vi "Panel Resized.vi"(6 "Sizing Refnums":T2, 8 "error in (no error)":errorcluster, 9 "Origin":cluster{"H":i16, "V":i16}, 10 "NewBnds":T1, 11 "Size Constraints":cluster{"min tab width":i32, "w/h":dbl}) -> (0 "error out":errorcluster)   [LabVIEW 2016]
uses:
  <vilib>/Utility/miscctls.llb/LVRectTypeDef.ctl
  <vilib>/Utility/miscctls.llb/LVRowAndColumnTypeDef.ctl
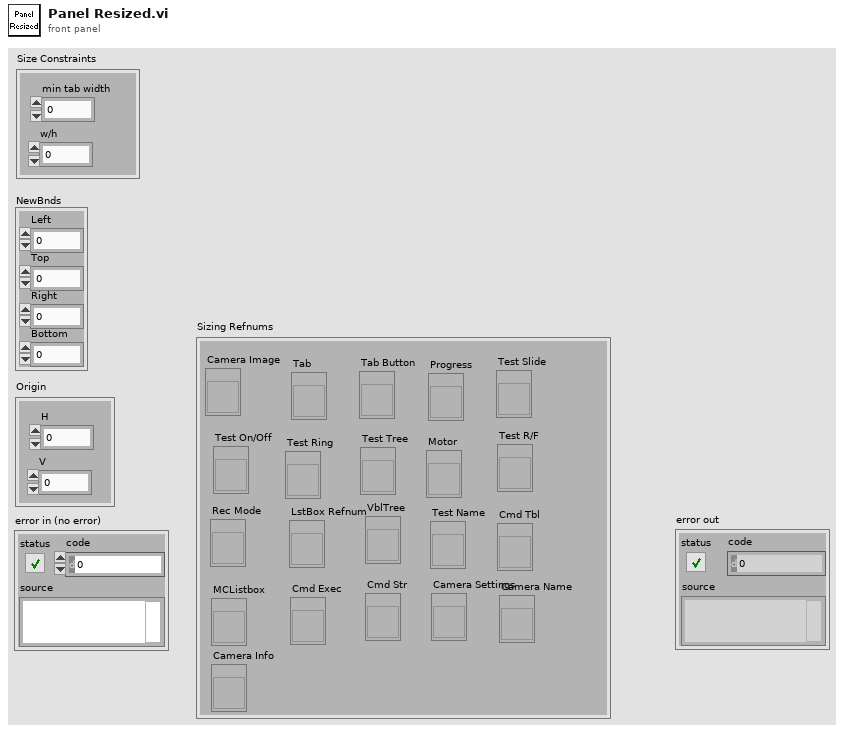
[diagram p1: front panel]
types:
  T1 = typedef "LVRectTypeDef.ctl" = cluster{"Left":i16, "Top":i16, "Right":i16, "Bottom":i16}
  T2 = cluster{"Camera Image":refnum<vi>, "Tab":refnum<vi>, "Tab Button":refnum<vi>, "Rec Mode":refnum<vi>, "Test Slide":refnum<vi>, "Test On/Off":refnum<vi>, "Test Ring":refnum<vi>, "Test R/F":refnum<vi>, "Test Name":refnum<vi>, "Motor":refnum<vi>, "Progress":refnum<vi>, "LstBox Refnum":refnum<vi>, "Test Tree":refnum<vi>, "VblTree":refnum<vi>, "Cmd Tbl":refnum<vi>, "MCListbox":refnum<vi>, "Cmd Exec":refnum<vi>, "Cmd Str":refnum<vi>, "Camera Settings":refnum<vi>, "Camera Name":refnum<vi>, "Camera Info":refnum<vi>}
  T3 = typedef "LVRowAndColumnTypeDef.ctl" = cluster{"Row":i32, "Column":i32}
  T4 = typedef "LVPositionTypeDef.ctl" = cluster{"Left":i32, "Top":i32}
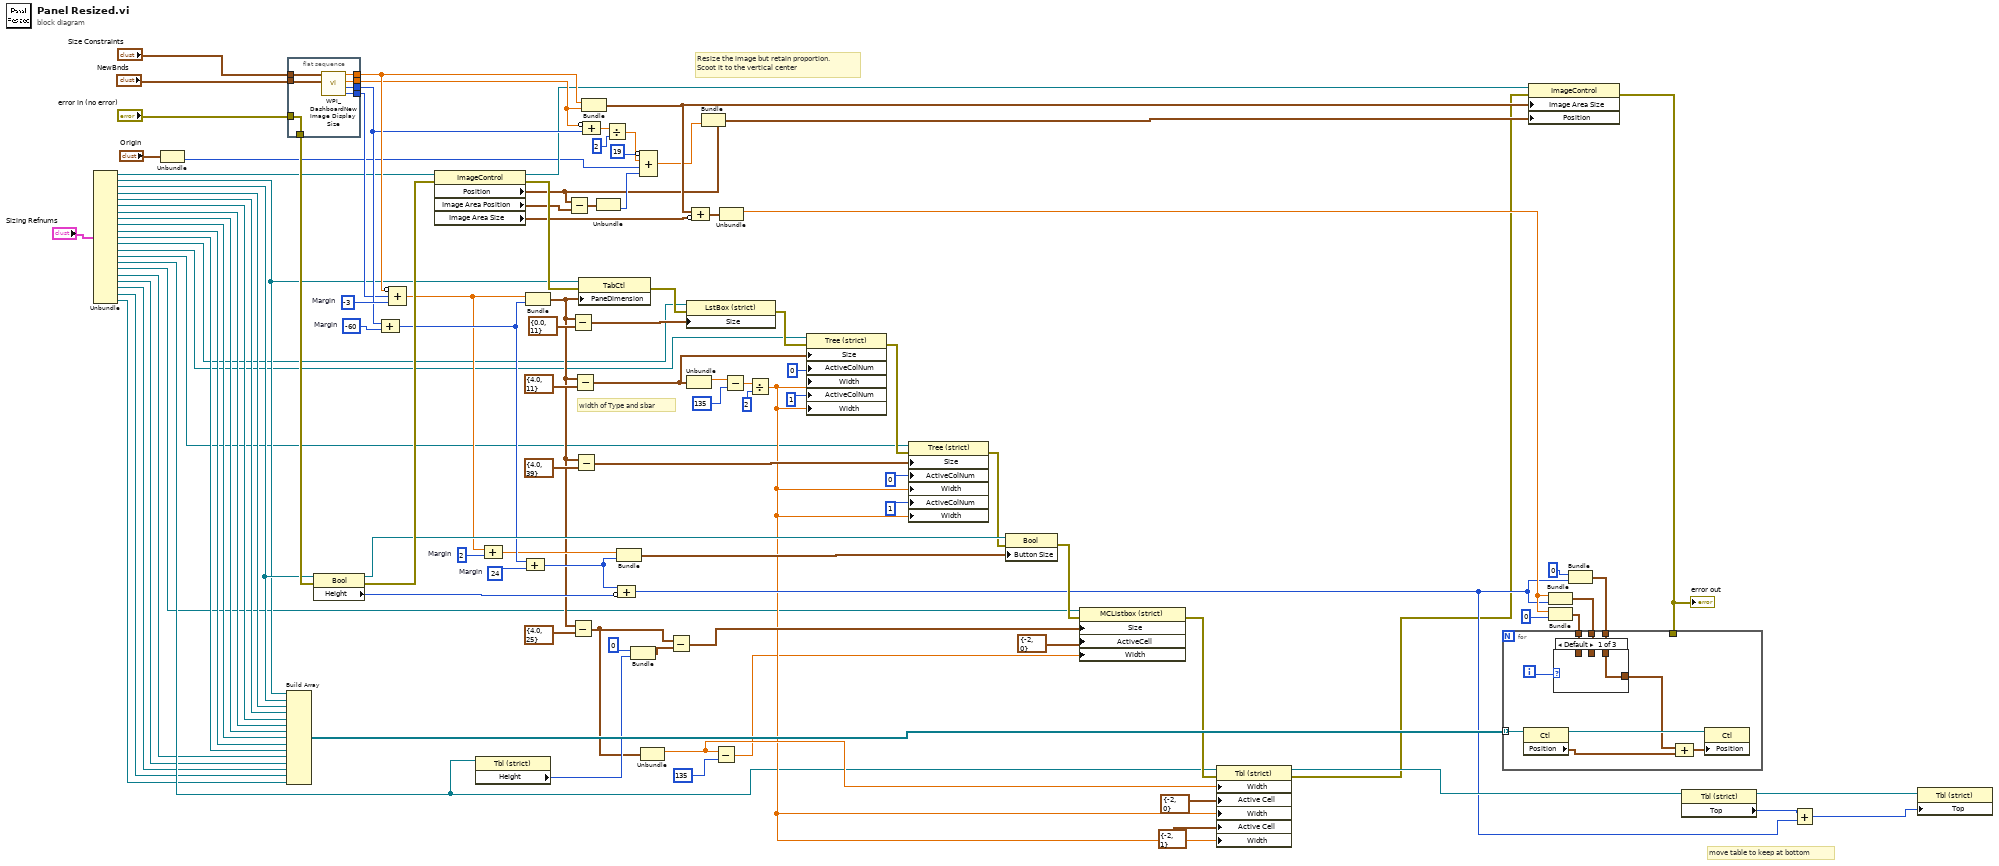
[diagram p0: block diagram]
diagram:
  w94 = 24  # Margin
  w92 = 2  # Margin
  w88 = -60  # Margin
  w98 = -3  # Margin
  # "move table to keep at bottom"
  # "width of Type and sbar"
  # "Resize the image but retain proportion.\nScoot it to the vertical center"
  n1 = Unbundle("Sizing Refnums") -> ("Camera Image"=w62:refnum<vi>, "Tab"=w63:refnum<vi>, "Tab Button"=w71:refnum<vi>, "Rec Mode"=w18:refnum<vi>, "Test Slide"=w17:refnum<vi>, "Test On/Off"=w16:refnum<vi>, "Test Ring"=w15:refnum<vi>, "Test R/F"=w14:refnum<vi>, "Test Name"=w13:refnum<vi>, "Motor"=w12:refnum<vi>, "Progress"=w11:refnum<vi>, "LstBox Refnum"=w10:refnum<vi>, "Test Tree"=w9:refnum<vi>, "VblTree"=w8:refnum<vi>, "Cmd Tbl"=w7:refnum<vi>, "MCListbox"=w6:refnum<vi>, "Cmd Exec"=w5:refnum<vi>, "Cmd Str"=w4:refnum<vi>, "Camera Settings"=w3:refnum<vi>, "Camera Name"=w2:refnum<vi>, "Camera Info"=w1:refnum<vi>)
  n2 = Unbundle("Origin") -> ("V"=w68:i16)  [unwired: 1 out]
  n3 = Build Array(w63, w71, w18, w17, w16, w15, w14, w13, w12, w11, w5, w4, w3, w2, w1) -> (w107:refnum<vi>[])
  n4 = flat-sequence {
    tunnel: "NewBnds" -> [w114]
    tunnel: "Size Constraints" -> [w113]
    tunnel: [w112] -> w87
    tunnel: [w111] -> w95
    tunnel: [w110] -> w96
    tunnel: [w109] -> w97
    tunnel: [w108] -> w106
    tunnel: "error in (no error)" -> [w108]
    frame #0 {
      n5 = call <vilib>:"WPI_DashboardNew Image Display Size.vi"("NewBnds"=w114, "Size Constraints"=w113) -> ("Window Width"=w112:i16, "Window Height"=w110:i16, "Height"=w111:dbl, "Width"=w109:dbl)  [unwired: 6 in]
    }
  }
  n6 = property class="Bool"(reference=w71, error in=w106) -> (reference out=w101:refnum<vi>, error out=w105:errorcluster, "Height"=w100:u32)
  n7 = Compound Arithmetic op=unknown(w96, w88) -> (w93:i32)
  n8 = Compound Arithmetic op=ADD(invert w97, w87, w98) -> (w91:dbl)
  n9 = property class="ImageControl"(reference=w62, error in=w105) -> (reference out=w80:refnum<vi>, error out=w104:errorcluster, "Position"=w79:T4, "Image Area Position"=w74:cluster{"Left":i32, "Top":i32}, "Image Area Size"=w85:cluster{"Width":u32, "Height":u32})
  n10 = property class="Tbl (strict)"(reference=w7) -> ("Height"=w37:u32)  [unwired: 1 in, 2 out]
  n11 = Compound Arithmetic op=ADD(w91, w92) -> (w90:dbl)
  n12 = Bundle(w91, w93) -> (w32:cluster{dbl, i32})  [unwired: 1 in]
  n13 = Compound Arithmetic op=ADD(w93, w94) -> (w99:i32)
  n14 = Subtract(x=w79, y=w74) -> (x-y=w81:T4)
  n15 = Subtract(x=w32, y=cluster{dbl, i32} {0.0, 11}) -> (x-y=w60:cluster{dbl, i32})
  n16 = Subtract(x=w32, y=cluster{dbl, i32} {4.0, 25}) -> (x-y=w34:cluster{dbl, i32})
  n17 = Subtract(x=w32, y=cluster{dbl, i32} {4.0, 11}) -> (x-y=w50:cluster{dbl, i32})
  n18 = Subtract(x=w32, y=cluster{dbl, i32} {4.0, 39}) -> (x-y=w56:cluster{dbl, i32})
  n19 = property class="TabCtl"(reference=w63, error in=w104, "PaneDimension"=w32) -> (error out=w61:errorcluster)  [unwired: 1 out]
  n20 = Bundle("Width"=w97, "Height"=w95) -> (w83:cluster{"Width":dbl, "Height":dbl})  [unwired: 1 in]
  n21 = Compound Arithmetic op=ADD(invert w95, w96) -> (w75:dbl)
  n22 = Unbundle(w81) -> ("Top"=w82:i32)  [unwired: 1 out]
  n23 = Divide(x=w75, y=2) -> (x/y=w77:dbl)
  n24 = Bundle(w90, w99) -> (w89:cluster{dbl, i32})  [unwired: 1 in]
  n25 = Compound Arithmetic op=ADD(w99, invert w100) -> (w28:u32)
  n26 = Bundle(0, "Height"=w37) -> (w35:cluster{i32, "Height":u32})  [unwired: 1 in]
  n27 = Compound Arithmetic op=ADD(invert 19, w77, w68, w82) -> (w78:dbl)
  n28 = Unbundle(w34) -> (w23:dbl)  [unwired: 1 out]
  n29 = Subtract(x=w34, y=w35) -> (x-y=w33:cluster{dbl, u32})
  n30 = property class="LstBox (strict)"(reference=w10, error in=w61, "Size"=w60) -> (error out=w55:errorcluster)  [unwired: 1 out]
  n31 = Unbundle(w50) -> (w49:dbl)  [unwired: 1 out]
  n32 = Compound Arithmetic op=ADD(w83, invert w85) -> (w86:cluster{"Width":dbl, "Height":dbl})
  n33 = Bundle(cluster=w79, "Top"=w78) -> (w84:T4)  [unwired: 1 in]
  n34 = Subtract(x=w23, y=135) -> (x-y=w20:dbl)
  n35 = Unbundle(w86) -> ("Width"=w102:dbl)  [unwired: 1 out]
  n36 = Subtract(x=w49, y=135 ("Active Cell:Active Column Number")) -> (x-y=w45:dbl)
  n37 = Divide(x=w45, y=2 ("Active Cell:Active Column Number")) -> (x/y=w21:dbl)
  n38 = property class="Tree (strict)"(reference=w9, error in=w55, "Size"=w50, "ActiveColNum"=0 ("Active Cell:Active Column Number"), "Width"=w21, "ActiveColNum"=1 ("Active Cell:Active Column Number"), "Width"=w21) -> (error out=w54:errorcluster)  [unwired: 1 out]
  n39 = property class="Tree (strict)"(reference=w8, error in=w54, "Size"=w56, "ActiveColNum"=0 ("Active Cell:Active Column Number"), "Width"=w21, "ActiveColNum"=1 ("Active Cell:Active Column Number"), "Width"=w21) -> (error out=w53:errorcluster)  [unwired: 1 out]
  n40 = property class="Bool"(reference=w101, error in=w53, "Button Size"=w89) -> (error out=w41:errorcluster)  [unwired: 1 out]
  n41 = property class="MCListbox (strict)"(reference=w6, error in=w41, "Size"=w33, "ActiveCell"=T3 {"Row"=-2, "Column"=0} ("Active Cell:Active Cell"), "Width"=w20) -> (error out=w38:errorcluster)  [unwired: 1 out]
  n42 = property class="Tbl (strict)"(reference=w7, error in=w38, "Width"=w23, "Active Cell"=T3 {"Row"=-2, "Column"=0} ("Active Cell:Active Cell"), "Width"=w21, "Active Cell"=T3 {"Row"=-2, "Column"=1} ("Active Cell:Active Cell"), "Width"=w21) -> (reference out=w31:refnum<vi>, error out=w26:errorcluster)
  n43 = property class="ImageControl"(reference=w80, error in=w26, "Image Area Size"=w83, "Position"=w84) -> (error out=w67:errorcluster)  [unwired: 1 out]
  "error out" <- w67
  n44 = Bundle("Width"=w102, w28) -> (w73:cluster{"Width":dbl, u32})  [unwired: 1 in]
  n45 = Bundle("Width"=w102, 0) -> (w72:cluster{"Width":dbl, i32})  [unwired: 1 in]
  n46 = Bundle(0, w28) -> (w42:cluster{i32, u32})  [unwired: 1 in]
  n47 = for {
    tunnel: w107 -> [w123] mode=indexing
    tunnel: w73 -> [w117]
    tunnel: w72 -> [w118]
    tunnel: w67 -> [_]
    tunnel: w42 -> [w116]
    i -> [w119]
    n48 = property class="Ctl"(reference=w123) -> (reference out=w122:refnum<vi>, "Position"=w121:T4)  [unwired: 1 in, 1 out]
    n49 = case shown="Default" w119 {
      tunnel: w118 -> [_ w125 _]
      tunnel: w117 -> [_ _ w126]
      tunnel: w116 -> [w124 _ _]
      tunnel: [w124 w125 w126] -> w115
      frame Default {
      }
      frame 0, 1 {
      }
      frame 2 {
      }
    }
    n50 = Compound Arithmetic op=ADD(w115, w121) -> (w120:cluster{dbl, u32})
    n51 = property class="Ctl"(reference=w122, "Position"=w120) -> ()  [unwired: 1 in, 2 out]
  }
  n52 = property class="Tbl (strict)"(reference=w31) -> (reference out=w30:refnum<vi>, "Top"=w29:i32)  [unwired: 1 in, 1 out]
  n53 = Add(x=w29, y=w28) -> (x+y=w27:u32)
  n54 = property class="Tbl (strict)"(reference=w30, "Top"=w27) -> ()  [unwired: 1 in, 2 out]
